vi "Begin.vi"(8 "error in":errorcluster) -> (0 "error out":errorcluster)   [LabVIEW 2019]
doc: "Called before other user functions, this VI is expected to open initial I/O refnums, load in file data, and do all program initialization. Notice that the <B>error out</B> terminal is simply used for data flow. Wiring it to other structures or subVIs ensures that this VI runs first."
uses:
  <vilib>/Rock Robotics/WPI/DriverStation/WPI_DriverStationRobotMode2.ctl
  <vilib>/Rock Robotics/WPI/Joystick/WPI_JoystickDeviceEnum.ctl
  <vilib>/Rock Robotics/SystemInterfaces/DIO/FPGA_DIOPWMChannel.ctl
  <vilib>/Rock Robotics/SystemInterfaces/DIO/FPGA_DIORelayChannel.ctl
  <vilib>/Rock Robotics/WPI/Solenoid/WPI_SolenoidChannel.ctl
  <vilib>/Rock Robotics/SystemInterfaces/DIO/FPGA_DIOChannel.ctl
  <vilib>/Rock Robotics/SystemInterfaces/i2clib/i2c_bus.ctl
  <vilib>/Rock Robotics/SystemInterfaces/AI/FPGA_AIChannel.ctl
  Robot Global Data.vi
  <vilib>/Rock Robotics/WPI/ThirdParty/Sensors/navX/_Processing Loop/FRIC_navX_Internal_SPI_ProcessingLoop.vi
  <vilib>/Rock Robotics/WPI/MotorControl/WPI_MotorControlOpen SPARK.vi
  <vilib>/Rock Robotics/WPI/MotorControl/WPI_MotorControlOpen Talon.vi
  <vilib>/Rock Robotics/WPI/Solenoid/WPI_SolenoidOpenSingle.vi
  <vilib>/Rock Robotics/WPI/Counter/WPI_CounterDigitalInputToDigitalSource.vi
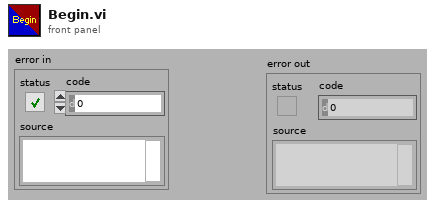
[diagram p1: front panel]
types:
  T1 = typedef "WPI_DriverStationRobotMode2.ctl" = enum16{"Autonomous Disabled", "Autonomous Enabled", "Teleop Disabled", "Teleop Enabled", "Disconnected", "Finish", "Test Disabled", "Test Enabled", "Emergency Stopped"}
  T2 = typedef "WPI_JoystickDeviceEnum.ctl" = enum16{"USB 0", "USB 1", "USB 2", "USB 3", "USB 4", "USB 5"}
  T3 = enum16{"FollowerType_PercentOutput", "FollowerType_AuxOutput1"}
  T4 = typedef "WPI_SolenoidChannel.ctl" = enum8{"Solenoid 0", "Solenoid 1", "Solenoid 2", "Solenoid 3", "Solenoid 4", "Solenoid 5", "Solenoid 6", "Solenoid 7", "Invalid"}
  T5 = typedef "FPGA_DIORelayChannel.ctl" = enum8{"Relay 0", "Relay 1", "Relay 2", "Relay 3", "Invalid"}
  T6 = typedef "FPGA_DIOPWMChannel.ctl" = enum8{"PWM 0", "PWM 1", "PWM 2", "PWM 3", "PWM 4", "PWM 5", "PWM 6", "PWM 7", "PWM 8", "PWM 9", "PWM MXP 0", "PWM MXP 1", "PWM MXP 2", "PWM MXP 3", "PWM MXP 4", "PWM MXP 5", "PWM MXP 6", "PWM MXP 7", "PWM MXP 8", "PWM MXP 9", "Invalid"}
  T7 = typedef "FPGA_AIChannel.ctl" = enum8{"AI 0", "AI 1", "AI 2", "AI 3", "AI MXP 0", "AI MXP 1", "AI MXP 2", "AI MXP 3", "Invalid"}
  T8 = typedef "i2c_bus.ctl" = enum16{"I2C On-Board", "I2C MXP", "Invalid"}
  T9 = typedef "WPI_CompressorDevRef.ctl" = cluster{"DevStatus":errorcluster, "Pneumatics Control Module":u8}
  T10 = typedef "WPI_JoystickDevRef.ctl" = cluster{"Device":T2}
  T11 = typedef "WPI_MotorControlDeviceRef.ctl" = cluster{"DeviceStatus":errorcluster, "Type":T12, "PWM":cluster{"PWM Channel":T6, "DeadBand":T13}, "CAN":cluster{"Device Number":u8, "SetOutput VI Ref":variant, "GetOutput VI Ref":variant, "Enable VI Ref":variant, "Disable VI Ref":variant, "Data":variant}, "Invert":bool, "DIO PWM":cluster{"PWM \"Enable\" Channel":T6, "DIOChannel":T14, "PWM Rate":dbl}}
  T12 = typedef "WPI_MotorControlType.ctl" = enum16{"PWM", "CAN", "DIO PWM"}
  T13 = typedef "WPI_PWMDeadband.ctl" = cluster{"Name":string, "maxPositivePwm":i32, "minPositivePwm":i32, "centerPwm":i32, "maxNegativePwm":i32, "minNegativePwm":i32, "angularRange":u16}
  T14 = typedef "FPGA_DIOChannel.ctl" = enum8{"DIO 0", "DIO 1", "DIO 2", "DIO 3", "DIO 4", "DIO 5", "DIO 6", "DIO 7", "DIO 8", "DIO 9", "DIO MXP 0", "DIO MXP 1", "DIO MXP 2", "DIO MXP 3", "DIO MXP 4", "DIO MXP 5", "DIO MXP 6", "DIO MXP 7", "DIO MXP 8", "DIO MXP 9", "DIO MXP 10", "DIO MXP 11", "DIO MXP 12", "DIO MXP 13", "DIO MXP 14", "DIO MXP 15", "SPI Port CS1", "SPI Port CS2", "SPI Port CS3", "SPI Port MISO", "SPI Port MOSI", "Invalid"}
  T15 = typedef "WPI_RelayDevRef.ctl" = cluster{"DevStatus":errorcluster, "Relay Channel":T5, "Relay Direction":T16}
  T16 = typedef "WPI_RelayDirection.ctl" = enum16{"Both directions", "Forward only", "Reverse only"}
  T17 = typedef "WPI_SolenoidDevRef.ctl" = cluster{"DevStatus":errorcluster, "Pneumatics Control Module":u8, "Forward Solenoid Channel":T4, "Reverse Solenoid Channel":T4}
  T18 = typedef "WPI_DigitalInputDevRef.ctl" = cluster{"DevStatus":errorcluster, "DIO Channel":T14}
  T19 = typedef "WPI_AnalogChannelDevRef.ctl" = cluster{"DevStatus":errorcluster, "Analog Channel":T7}
  T20 = typedef "FPGA_CounterEncoderSourceConvertionLVSourceType.ctl" = cluster{"DevStatus":errorcluster, "AnalogTriggerMode?":bool, "DigitalMode":cluster{"DIO Channel":T21}, "AnalogTriggerMode":cluster{"AnalogTriggerIndex":T22, "OutputType":T23}}
  T21 = typedef "FPGA_DIODigitalSourceChannel.ctl" = enum8{"DIO 0", "DIO 1", "DIO 2", "DIO 3", "DIO 4", "DIO 5", "DIO 6", "DIO 7", "DIO 8", "DIO 9", "DIO MXP 0", "DIO MXP 1", "DIO MXP 2", "DIO MXP 3", "DIO MXP 4", "DIO MXP 5", "DIO MXP 6", "DIO MXP 7", "DIO MXP 8", "DIO MXP 9", "DIO MXP 10", "DIO MXP 11", "DIO MXP 12", "DIO MXP 13", "DIO MXP 14", "DIO MXP 15", "SPI Port CS1", "SPI Port CS2", "SPI Port CS3", "SPI Port MISO", "SPI Port MOSI", "Disabled"}
  T22 = typedef "FPGA_AnalogTriggerIndex.ctl" = enum8{"Trig 0", "Trig 1", "Trig 2", "Trig 3", "Trig 4", "Trig 5", "Trig 6", "Trig 7", "Invalid"}
  T23 = typedef "FPGA_AnalogTriggerOutType.ctl" = enum16{"InWindow", "TriggerState", "Rising", "Falling"}
  T24 = typedef "Color Sensor V3 DevRef.ctl" = cluster{"I2CDevRef":T25}
  T25 = typedef "WPI_I2CDevRef.ctl" = cluster{"DevStatus":errorcluster, "Device Address":u8, "Handle":i32, "I2C Bus":T8}
  T26 = typedef "WPI_EncoderDevRef.ctl" = cluster{"DevStatus":errorcluster, "EncoderIndex":T27, "CounterIndex":T28, "DistancePerCount":dbl, "Decoding Type":T29}
  T27 = typedef "FPGA_EncoderIdx.ctl" = enum8{"Enc 0", "Enc 1", "Enc 2", "Enc 3", "Enc 4", "Enc 5", "Enc 6", "Enc 7", "Invalid"}
  T28 = typedef "FPGA_CounterCtrSystemIndex.ctl" = enum8{"Ctr 0", "Ctr 1", "Ctr 2", "Ctr 3", "Ctr 4", "Ctr 5", "Ctr 6", "Ctr 7", "Invalid"}
  T29 = typedef "WPI_EncoderType.ctl" = enum16{"1x", "2x", "4x"}
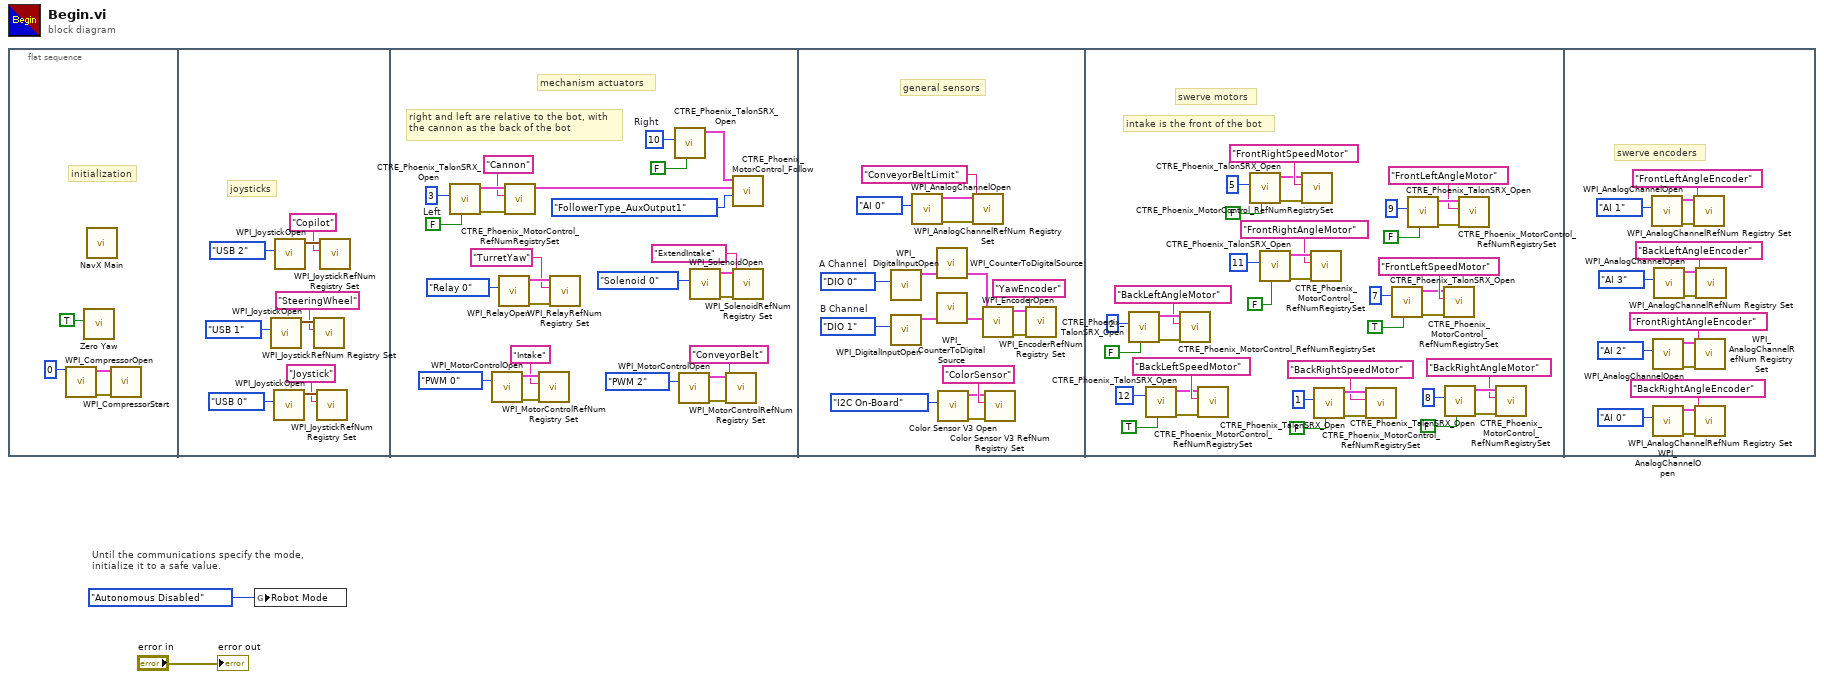
[diagram p0: block diagram]
diagram:
  # "Until the communications specify the mode,\ninitialize it to a safe value."
  n1 = flat-sequence {
    frame #0 {
      # "initialization"
      n2 = call <vilib>:"WPI_CompressorOpen.vi"("Pneumatics Control Module (0)"=u8 0) -> ("CompressorDevRef"=w3:T9, "error out"=w6:errorcluster)  [unwired: 13 in]
      n3 = call <vilib>:"Zero Yaw.vi"("Zero"=TRUE) -> ()  [unwired: 11 in]
      n4 = call-poly <vilib>:"NavX Main.vi"() -> ()  [unwired: 12 in]
      n5 = call <vilib>:"WPI_CompressorStart.vi"("error in (no error)"=w6, "CompressorDevRef"=w3) -> ()  [unwired: 8 in, 2 out]
    }
    frame #1 {
      # "joysticks"
      n6 = call <vilib>:"WPI_JoystickOpen.vi"("JoystickDevice"=WPI_JoystickDeviceEnum."USB 1") -> ("JoystickDevRef"=w11:T10)  [unwired: 10 in]
      n7 = call <vilib>:"WPI_JoystickOpen.vi"("JoystickDevice"=WPI_JoystickDeviceEnum."USB 0") -> ("JoystickDevRef"=w12:T10)  [unwired: 10 in]
      n8 = call <vilib>:"WPI_JoystickOpen.vi"("JoystickDevice"=WPI_JoystickDeviceEnum."USB 2") -> ("JoystickDevRef"=w15:T10)  [unwired: 10 in]
      n9 = call <vilib>:"WPI_JoystickRefNum Registry Set.vi"("refnum name"="SteeringWheel", "JoystickDevRef"=w11) -> ()  [unwired: 8 in, 2 out]
      n10 = call <vilib>:"WPI_JoystickRefNum Registry Set.vi"("refnum name"="Joystick", "JoystickDevRef"=w12) -> ()  [unwired: 8 in, 2 out]
      n11 = call <vilib>:"WPI_JoystickRefNum Registry Set.vi"("refnum name"="Copilot", "JoystickDevRef"=w15) -> ()  [unwired: 8 in, 2 out]
    }
    frame #2 {
      w32 = u8 3  # Left
      w33 = u8 10  # Right
      # "right and left are relative to the bot, with\nthe cannon as the back of the bot"
      # "mechanism actuators"
      n12 = call <vilib>:"CTRE_Phoenix_TalonSRX_Open.vi"("Invert"=FALSE, "Device Number"=w32) -> ("error out"=w20:errorcluster, "CAN Talon SRX Ref"=w21:T11)  [unwired: 8 in]
      n13 = call-poly <vilib>:"WPI_MotorControlOpen.vi"("PWM Channel"=FPGA_DIOPWMChannel."PWM 0") -> ("error out"=w41:errorcluster, "MotorControlDeviceRef"=w40:T11)  [unwired: 9 in]
      n14 = call <vilib>:"WPI_RelayOpen.vi"("Relay Channel"=FPGA_DIORelayChannel."Relay 0") -> ("error out"=w31:errorcluster, "RelayDevRef"=w30:T15)  [unwired: 9 in]
      n15 = call <vilib>:"CTRE_Phoenix_MotorControl_RefNumRegistrySet.vi"("error in (no error)"=w20, "refnum name"="Cannon", "PhoenixMotorControlDevRef"=w21) -> ("PhoenixMotorControlDevRef"=w17:T11)  [unwired: 7 in, 1 out]
      n16 = call <vilib>:"WPI_MotorControlRefNum Registry Set.vi"("error in (no error)"=w41, "refnum name"="Intake", "MotorControlDevRef"=w40) -> ()  [unwired: 7 in, 2 out]
      n17 = call <vilib>:"WPI_RelayRefNum Registry Set.vi"("error in (no error)"=w31, "refnum name"="TurretYaw", "RelayDevRef"=w30) -> ()  [unwired: 7 in, 2 out]
      n18 = call <vilib>:"CTRE_Phoenix_TalonSRX_Open.vi"("Invert"=FALSE, "Device Number"=w33) -> ("CAN Talon SRX Ref"=w18:T11)  [unwired: 8 in, 1 out]
      n19 = call-poly <vilib>:"WPI_MotorControlOpen.vi"("PWM Channel"=FPGA_DIOPWMChannel."PWM 2") -> ("error out"=w37:errorcluster, "MotorControlDeviceRef"=w36:T11)  [unwired: 9 in]
      n20 = call-poly <vilib>:"WPI_SolenoidOpen.vi"("Solenoid Channel"=WPI_SolenoidChannel."Solenoid 0") -> ("error out"=w26:errorcluster, "SolenoidDevRef"=w27:T17)  [unwired: 9 in]
      n21 = call <vilib>:"WPI_MotorControlRefNum Registry Set.vi"("error in (no error)"=w37, "refnum name"="ConveyorBelt", "MotorControlDevRef"=w36) -> ()  [unwired: 7 in, 2 out]
      n22 = call <vilib>:"CTRE_Phoenix_MotorControl_Follow.vi"("FollowerType"=T3."FollowerType_AuxOutput1", "Master Controller to Follow"=w17, "PhoenixMotorControlDevRef"=w18) -> ()  [unwired: 7 in, 2 out]
      n23 = call <vilib>:"WPI_SolenoidRefNum Registry Set.vi"("error in (no error)"=w26, "refnum name"="ExtendIntake", "SolenoidDevRef"=w27) -> ()  [unwired: 7 in, 2 out]
    }
    frame #3 {
      w58 = FPGA_DIOChannel."DIO 1"  # B Channel
      w57 = FPGA_DIOChannel."DIO 0"  # A Channel
      # "general sensors"
      n24 = call <vilib>:"WPI_DigitalInputOpen.vi"("DIO Channel"=w57) -> ("DigitalInputDevRef"=w54:T18)  [unwired: 1 in, 9 out]
      n25 = call <vilib>:"WPI_DigitalInputOpen.vi"("DIO Channel"=w58) -> ("DigitalInputDevRef"=w55:T18)  [unwired: 1 in, 9 out]
      n26 = call <vilib>:"WPI_AnalogChannelOpen.vi"("Analog Channel"=FPGA_AIChannel."AI 0") -> ("error out"=w44:errorcluster, "AIDeviceRef"=w43:T19)  [unwired: 9 in]
      n27 = call-poly <vilib>:"WPI_CounterToDigitalSource.vi"("DigitalInputDevRef"=w54) -> ("Digital Source"=w53:T20)  [unwired: 6 out]
      n28 = call-poly <vilib>:"WPI_CounterToDigitalSource.vi"("DigitalInputDevRef"=w55) -> ("Digital Source"=w56:T20)  [unwired: 6 out]
      n29 = call <vilib>:"Color Sensor V3 Open.vi"("I2C Bus"=i2c_bus."I2C On-Board") -> ("error out"=w48:errorcluster, "ColorSensorDevRef"=w47:T24)  [unwired: 9 in]
      n30 = call <vilib>:"WPI_AnalogChannelRefNum Registry Set.vi"("error in (no error)"=w44, "refnum name"="ConveyorBeltLimit", "AIDeviceRef"=w43) -> ()  [unwired: 7 in, 2 out]
      n31 = call <vilib>:"WPI_EncoderOpen.vi"("BSource"=w56, "ASource"=w53) -> ("error out"=w52:errorcluster, "EncoderDevRef"=w51:T26)  [unwired: 6 in, 2 out]
      n32 = call <vilib>:"Color Sensor V3 RefNum Registry Set.vi"("error in (no error)"=w48, "refnum name"="ColorSensor", "ColorSensorDevRef"=w47) -> ()  [unwired: 7 in, 2 out]
      n33 = call <vilib>:"WPI_EncoderRefNum Registry Set.vi"("error in (no error)"=w52, "refnum name"="YawEncoder", "EncoderDevRef"=w51) -> ()  [unwired: 7 in, 2 out]
    }
    frame #4 {
      # "intake is the front of the bot"
      # "swerve motors"
      n34 = call <vilib>:"CTRE_Phoenix_TalonSRX_Open.vi"("Invert"=FALSE, "Device Number"=u8 2) -> ("error out"=w78:errorcluster, "CAN Talon SRX Ref"=w77:T11)  [unwired: 8 in]
      n35 = call <vilib>:"CTRE_Phoenix_TalonSRX_Open.vi"("Invert"=TRUE, "Device Number"=u8 12) -> ("error out"=w93:errorcluster, "CAN Talon SRX Ref"=w94:T11)  [unwired: 8 in]
      n36 = call <vilib>:"CTRE_Phoenix_MotorControl_RefNumRegistrySet.vi"("error in (no error)"=w78, "refnum name"="BackLeftAngleMotor", "PhoenixMotorControlDevRef"=w77) -> ()  [unwired: 7 in, 2 out]
      n37 = call <vilib>:"CTRE_Phoenix_MotorControl_RefNumRegistrySet.vi"("error in (no error)"=w93, "refnum name"="BackLeftSpeedMotor", "PhoenixMotorControlDevRef"=w94) -> ()  [unwired: 7 in, 2 out]
      n38 = call <vilib>:"CTRE_Phoenix_TalonSRX_Open.vi"("Invert"=FALSE, "Device Number"=u8 5) -> ("error out"=w82:errorcluster, "CAN Talon SRX Ref"=w83:T11)  [unwired: 8 in]
      n39 = call <vilib>:"CTRE_Phoenix_TalonSRX_Open.vi"("Invert"=FALSE, "Device Number"=u8 11) -> ("error out"=w66:errorcluster, "CAN Talon SRX Ref"=w65:T11)  [unwired: 8 in]
      n40 = call <vilib>:"CTRE_Phoenix_MotorControl_RefNumRegistrySet.vi"("error in (no error)"=w82, "refnum name"="FrontRightSpeedMotor", "PhoenixMotorControlDevRef"=w83) -> ()  [unwired: 7 in, 2 out]
      n41 = call <vilib>:"CTRE_Phoenix_MotorControl_RefNumRegistrySet.vi"("error in (no error)"=w66, "refnum name"="FrontRightAngleMotor", "PhoenixMotorControlDevRef"=w65) -> ()  [unwired: 7 in, 2 out]
      n42 = call <vilib>:"CTRE_Phoenix_TalonSRX_Open.vi"("Invert"=FALSE, "Device Number"=u8 1) -> ("error out"=w84:errorcluster, "CAN Talon SRX Ref"=w85:T11)  [unwired: 8 in]
      n43 = call <vilib>:"CTRE_Phoenix_MotorControl_RefNumRegistrySet.vi"("error in (no error)"=w84, "refnum name"="BackRightSpeedMotor", "PhoenixMotorControlDevRef"=w85) -> ()  [unwired: 7 in, 2 out]
      n44 = call <vilib>:"CTRE_Phoenix_TalonSRX_Open.vi"("Invert"=TRUE, "Device Number"=u8 7) -> ("error out"=w91:errorcluster, "CAN Talon SRX Ref"=w92:T11)  [unwired: 8 in]
      n45 = call <vilib>:"CTRE_Phoenix_TalonSRX_Open.vi"("Invert"=FALSE, "Device Number"=u8 9) -> ("error out"=w76:errorcluster, "CAN Talon SRX Ref"=w75:T11)  [unwired: 8 in]
      n46 = call <vilib>:"CTRE_Phoenix_MotorControl_RefNumRegistrySet.vi"("error in (no error)"=w91, "refnum name"="FrontLeftSpeedMotor", "PhoenixMotorControlDevRef"=w92) -> ()  [unwired: 7 in, 2 out]
      n47 = call <vilib>:"CTRE_Phoenix_TalonSRX_Open.vi"("Invert"=FALSE, "Device Number"=u8 8) -> ("error out"=w68:errorcluster, "CAN Talon SRX Ref"=w67:T11)  [unwired: 8 in]
      n48 = call <vilib>:"CTRE_Phoenix_MotorControl_RefNumRegistrySet.vi"("error in (no error)"=w76, "refnum name"="FrontLeftAngleMotor", "PhoenixMotorControlDevRef"=w75) -> ()  [unwired: 7 in, 2 out]
      n49 = call <vilib>:"CTRE_Phoenix_MotorControl_RefNumRegistrySet.vi"("error in (no error)"=w68, "refnum name"="BackRightAngleMotor", "PhoenixMotorControlDevRef"=w67) -> ()  [unwired: 7 in, 2 out]
    }
    frame #5 {
      # "swerve encoders"
      n50 = call <vilib>:"WPI_AnalogChannelOpen.vi"("Analog Channel"=FPGA_AIChannel."AI 1") -> ("error out"=w113:errorcluster, "AIDeviceRef"=w114:T19)  [unwired: 9 in]
      n51 = call <vilib>:"WPI_AnalogChannelOpen.vi"("Analog Channel"=FPGA_AIChannel."AI 2") -> ("error out"=w105:errorcluster, "AIDeviceRef"=w106:T19)  [unwired: 9 in]
      n52 = call <vilib>:"WPI_AnalogChannelOpen.vi"("Analog Channel"=FPGA_AIChannel."AI 0") -> ("error out"=w101:errorcluster, "AIDeviceRef"=w102:T19)  [unwired: 9 in]
      n53 = call <vilib>:"WPI_AnalogChannelOpen.vi"("Analog Channel"=FPGA_AIChannel."AI 3") -> ("error out"=w109:errorcluster, "AIDeviceRef"=w110:T19)  [unwired: 9 in]
      n54 = call <vilib>:"WPI_AnalogChannelRefNum Registry Set.vi"("error in (no error)"=w113, "refnum name"="FrontLeftAngleEncoder", "AIDeviceRef"=w114) -> ()  [unwired: 7 in, 2 out]
      n55 = call <vilib>:"WPI_AnalogChannelRefNum Registry Set.vi"("error in (no error)"=w105, "refnum name"="FrontRightAngleEncoder", "AIDeviceRef"=w106) -> ()  [unwired: 7 in, 2 out]
      n56 = call <vilib>:"WPI_AnalogChannelRefNum Registry Set.vi"("error in (no error)"=w101, "refnum name"="BackRightAngleEncoder", "AIDeviceRef"=w102) -> ()  [unwired: 7 in, 2 out]
      n57 = call <vilib>:"WPI_AnalogChannelRefNum Registry Set.vi"("error in (no error)"=w109, "refnum name"="BackLeftAngleEncoder", "AIDeviceRef"=w110) -> ()  [unwired: 7 in, 2 out]
    }
  }
  n58 = global write "Robot Global Data.vi" "Robot Mode"(WPI_DriverStationRobotMode2."Autonomous Disabled" ("Robot Mode")) -> ()
  "error out" <- "error in"
